vi "WIRE_CLEAN_3 (SubVI).vi"(6 "Steps":dbl, 9 "Final Value":dbl, 10 "Initial Value":dbl, 11 "VISA Refnum in":refnum<visa-resource-name>) -> (0 "error out":errorcluster, 1 "Numeric 3":dbl, 2 "Numeric":u32, 3 "VISA Refnum out":refnum<visa-resource-name>, 5 "Numeric 2":dbl)   [LabVIEW 2020]
uses:
  Program Files/National Instruments/LabVIEW 2020/instr.lib/Agilent B2900 Series/Agilent B2900 Series.lvlib
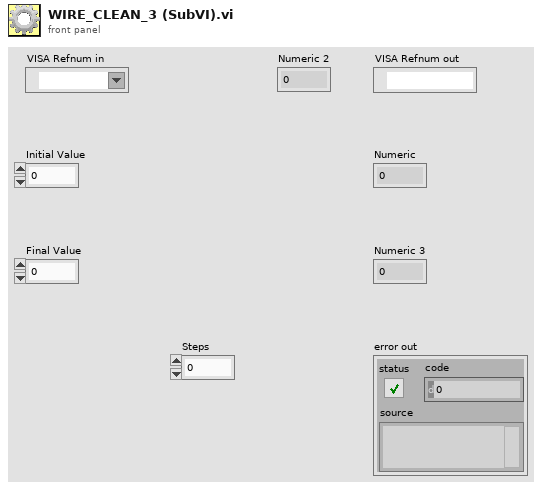
[diagram p1: front panel]
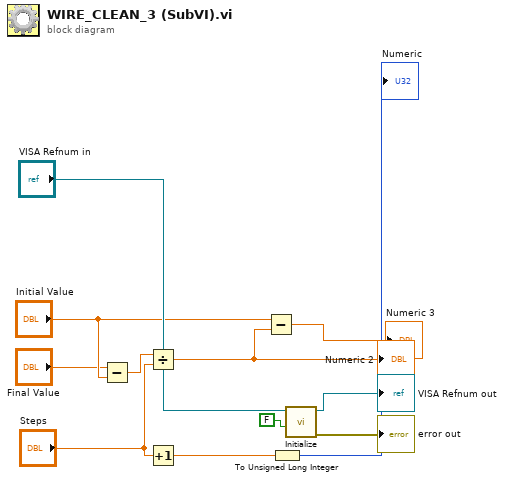
[diagram p0: block diagram]
diagram:
  n1 = Subtract(x="Final Value", y="Initial Value") -> (x-y=w3:dbl)
  n2 = Divide(x=w3, y="Steps") -> (x/y=w4:dbl)
  "Numeric 2" <- w4
  n3 = Increment(x="Steps") -> (x+1=w11:dbl)
  n4 = Subtract(x="Initial Value", y=w4) -> (x-y=→"Numeric 3":dbl)
  n5 = To Unsigned Long Integer(number=w11) -> (unsigned 32bit integer=→"Numeric":u32)
  n6 = call "Initialize.vi"("Reset (True)"=FALSE, "VISA resource name"="VISA Refnum in") -> ("error out"=→"error out":errorcluster, "VISA resource name out"=→"VISA Refnum out":refnum<visa-resource-name>)  [unwired: 8 in]
